vi "DP I-O Main Panel.vi"(11 "Expt State (in)":T2) -> (3 "State":T2)   [LabVIEW 2020]
uses:
  Typedefs/DP Stimulus Params.ctl
  epl-vi-lib/Utility VIs/Type Defs/Left-Right ring.ctl
  CFTS Main Panel SubVIs/CFTS-Experiment State.ctl
  Typedefs/DP-StimGen.ctl
  Typedefs/DP-Rejection Settings.ctl
  Typedefs/DP-Advanced Options.ctl
  CFTS Main Panel SubVIs/CFTS-Data Type Enum.ctl
panel:
  in  "Last user":string
  in  "Recalibrate":bool
  in  "Probe Mic Gain (dB)":dbl
  in  "Save Waves?":bool=TRUE
  out "User":string
  out "Run #":u16=14
  out "ID #":u16=1
  in  "Avg specs":T1={"# Time avgs "=8, "# Spectrum avgs"=4}
  out "Path":path
  in  "DP Params":T3={"Start (dB)"=20.0, "Stop (dB)"=70.0, "Step (dB)"=10.0, "Ear"=enum."Right", "Mode"=enum."L1 = L2 + 10 dB", "f2 freqs (kHz)"="5.6;8.0;11.3;16;22.6;32;"}
  out "advanced":bool
  in  "Advanced options":T5
  in  "Start":bool
  in  "Stop":bool
  out "exit signal":bool
  out "Error":bool
  in  "Reject":T6 caption="Rejection"
  in  "StimGen":T7={"Sampling Rate (Hz)"=200000.0, "Npts"=10000, "Data Folder"=path "", "Acoustic System"="", "Recalibrate?"=FALSE, "AO Channels"=[], "Mic  gain (dB)"=0.0, "F1, F2 speakers"=[], "Override recal check"=FALSE}
  out "Freqs":cluster{"f1":dbl, "f2":dbl, "2f1-f2":dbl}={"f1"=9419.759114583332, "f2"=11291.50390625, "2f1-f2"=7548.014322916664} {"2f1-f2" format="%.3f"; "f1" format="%.3f"; "f2" format="%.3f"}
  out "Abort":bool
  out "running":bool
  out "DP window":cluster{i32, "df (Hz)":dbl, dbl[]}(graph)={0, "df (Hz)"=0.02, []}
  out "I-O Plot":cluster{cluster{dbl, dbl}[]}[](graph)
  in  "Notes":string
  out "Full Spectrum":cluster{i32, "Freq Resolution":dbl, dbl[]}(graph)={0, "Freq Resolution"=20.345052083333332, []}
  in  "RETURN":bool
  # "Stimulus"
  # "Averaging"
  # "Response"
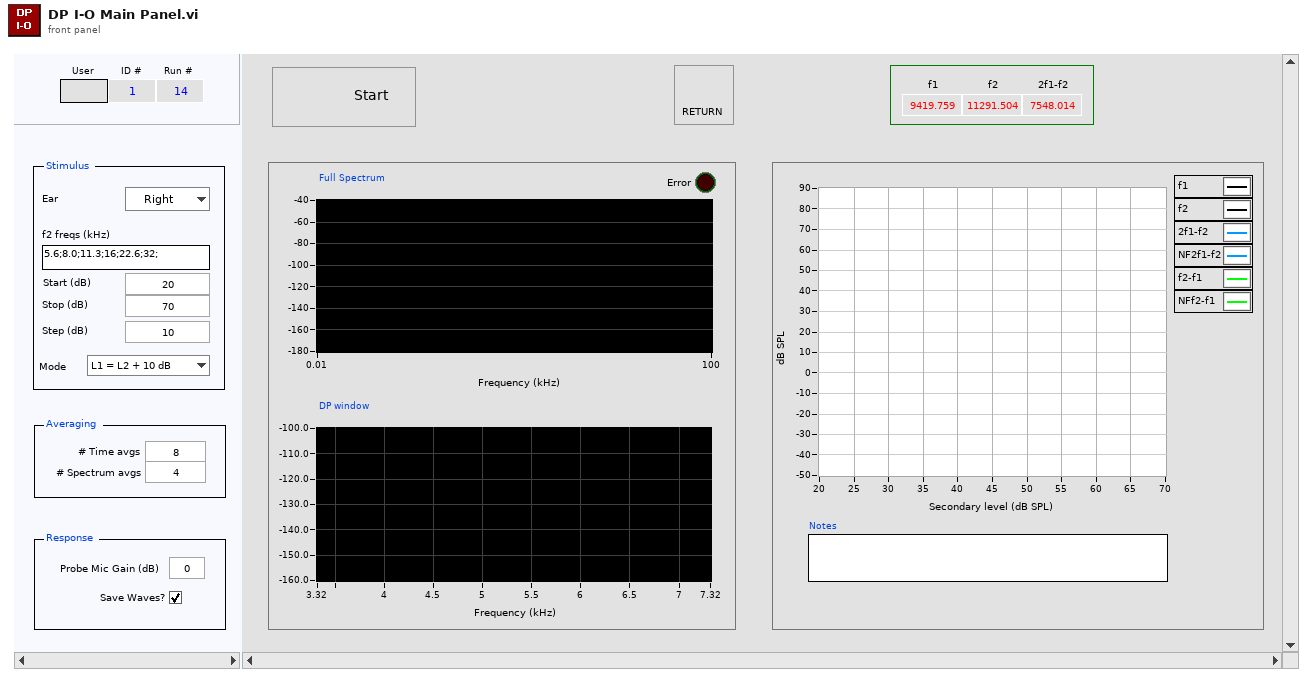
[diagram p1: front panel]
types:
  T1 = cluster{"# Time avgs ":i32, "# Spectrum avgs":i32}
  T2 = typedef "CFTS-Experiment State.ctl" = cluster{"Experimenter":string, "Number":u32, "Right":string, "Left":string, "Data Folder":path, "State File":path, "Version Info":string, "End Exposure Time":dbl, "Exposure Duration":string, "Run #":cluster{"CAP":i16, "ABR":i16, "DP":i16, "VsEP":i16, "MeasSeq":i16, "SubSeq":i16, "SFOAE":i16}}
  T3 = typedef "DP Stimulus Params.ctl" = cluster{"Start (dB)":dbl, "Stop (dB)":dbl, "Step (dB)":dbl, "Ear":T4, "Mode":enum16{"L1 = L2", "L1 = L2 + 10 dB"}, "f2 freqs (kHz)":string}
  T4 = typedef "Left-Right ring.ctl" = enum16{"Right", "Left"}
  T5 = typedef "DP-Advanced Options.ctl" = cluster{"TimeAvgExpr":string, "FreqAvgExpr":string}
  T6 = typedef "DP-Rejection Settings.ctl" = cluster{"Override":bool, "dB re 2f1-f2":dbl, "Min (dB SPL)":dbl}
  T7 = typedef "DP-StimGen.ctl" = cluster{"Sampling Rate (Hz)":dbl, "Npts":i32, "Data Folder":path, "Acoustic System":string, "Recalibrate?":bool, "AO Channels":i32[], "Mic  gain (dB)":dbl, "F1, F2 speakers":i32[], "Override recal check":bool}
  T8 = typedef "CFTS-Data Type Enum.ctl" = enum16{"CAP", "ABR", "DP", "VsEP", "MeasSeq", "SFOAE"}
  T9 = typedef "DP-Freqs.ctl" = cluster{"f1":dbl, "f2":dbl, "2f1-f2":dbl}
  T10 = typedef "DP-DataAcq.ctl" = cluster{"#spectra avgs":i32[], "#time avgs":i32[], "dt (ms)":dbl, "df (kHz)":dbl, "Npts":i32, "Save waves?":bool, "Data File":path, "AI Channels":u16[], "Sampling rate (Hz)":dbl, "Probe Tube Sensitivity":cluster{"Frequency":dbl[], "Mag":dbl[]}, "Mic gain (dB)":dbl, "ptIndex":i32}
  T11 = typedef "CFTS-Options.ctl" = cluster{"DP Artifact Rejection":bool, "Monitor vital signs ":bool, "Extension":string}
  T12 = cluster{"Shift":bool, "Ctrl":bool, "Alt":bool, "Cmd":bool, "Opt":bool}
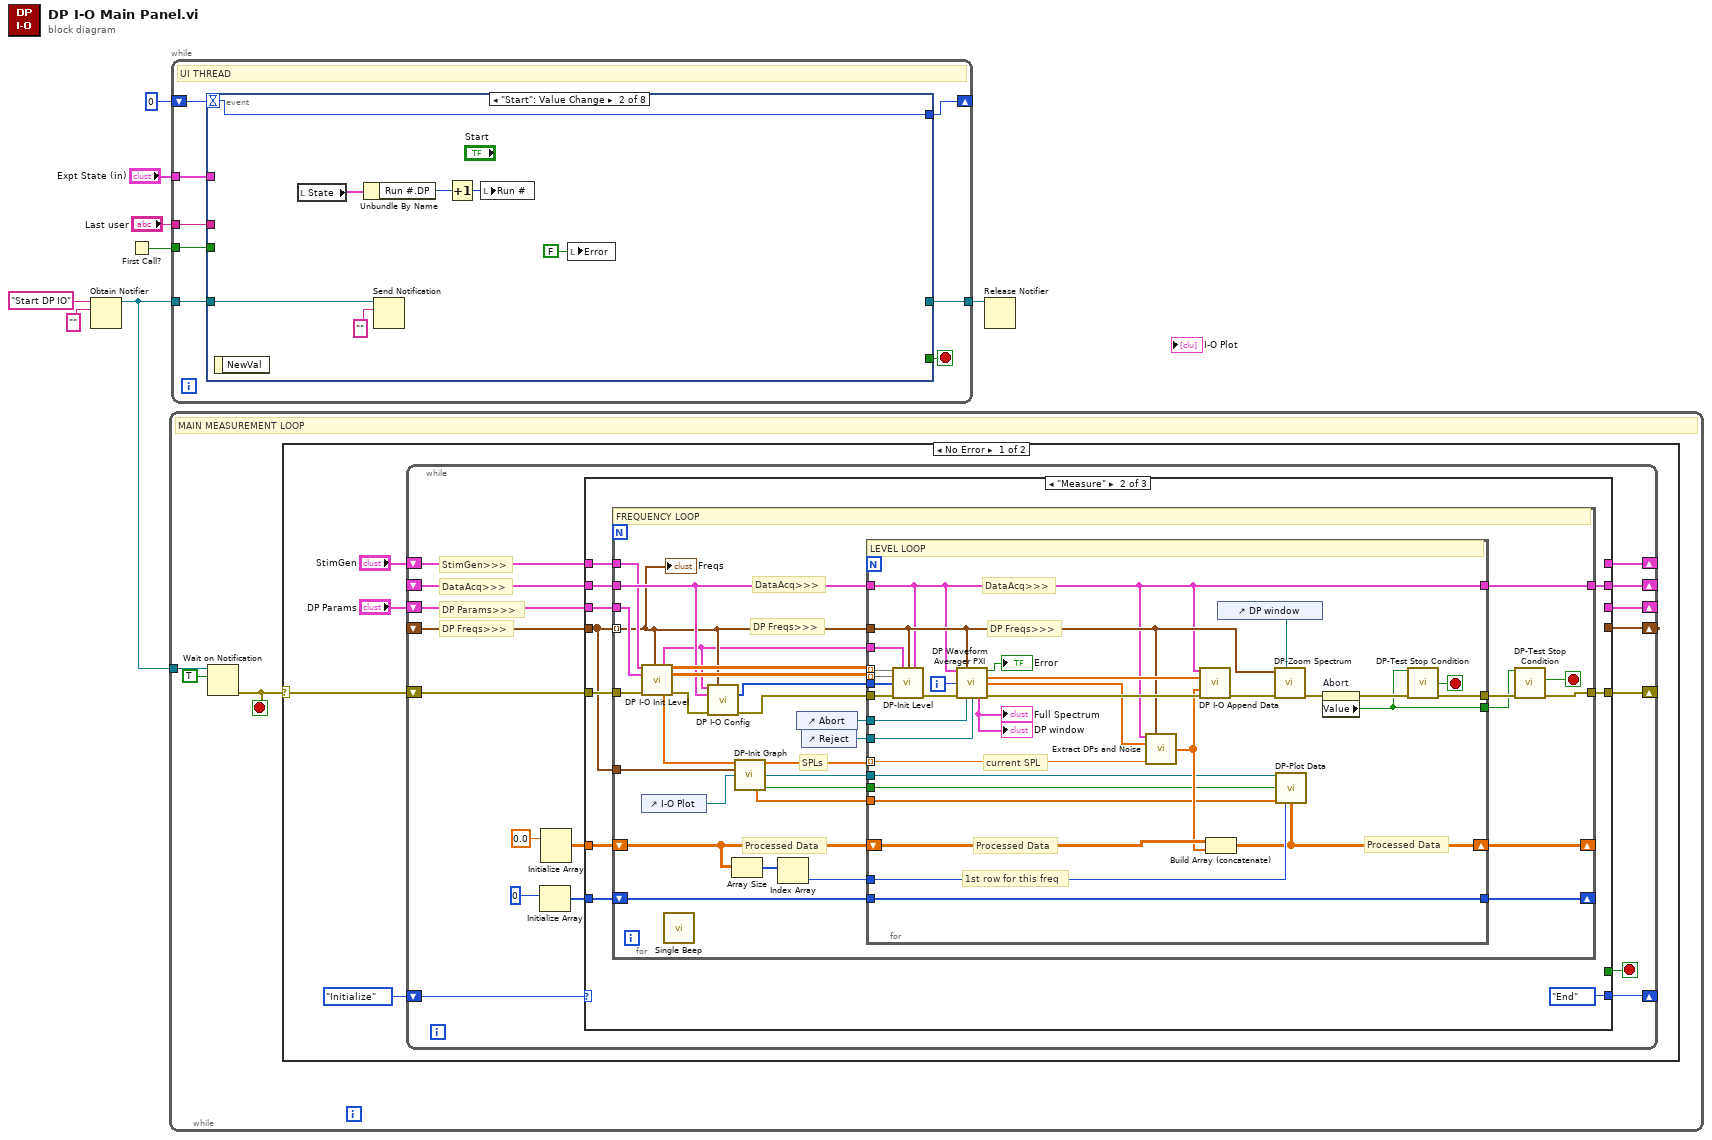
[diagram p0: block diagram]
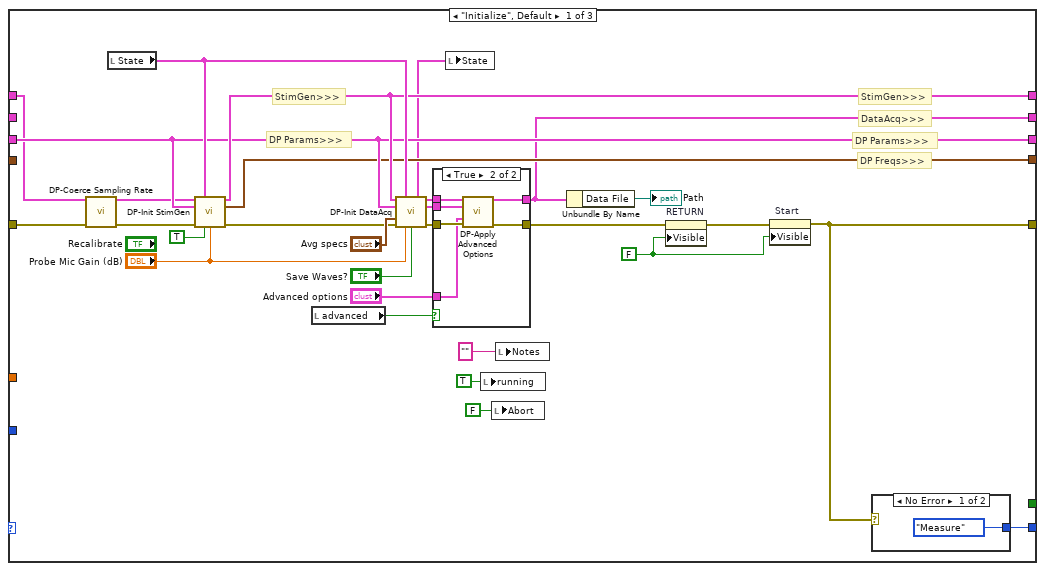
[diagram p2: hidden frame]
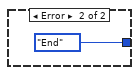
[diagram p4: hidden frame]
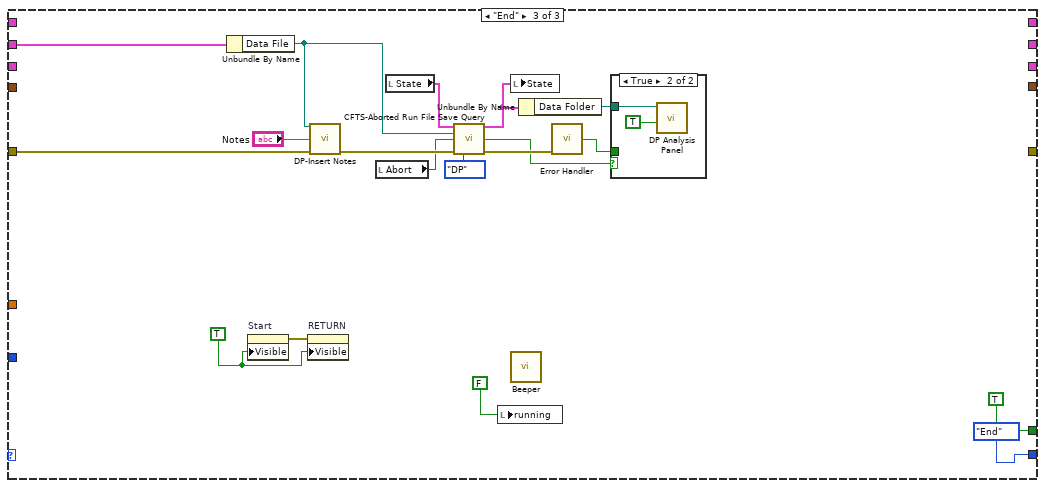
[diagram p5: hidden frame]
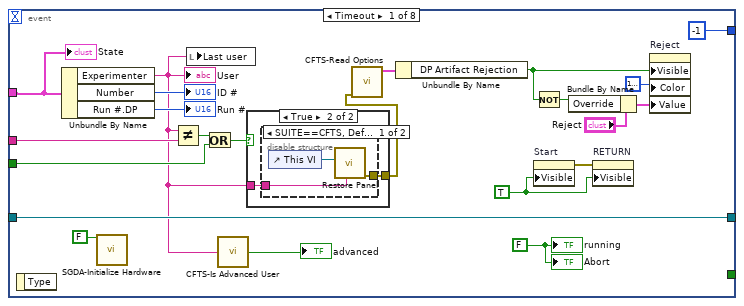
[diagram p8: hidden frame]
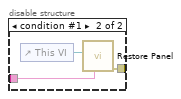
[diagram p10: hidden frame]
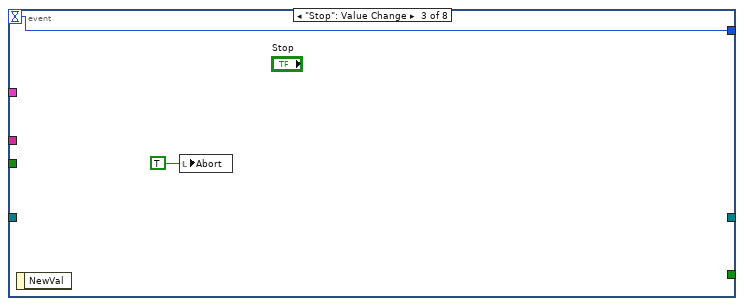
[diagram p11: hidden frame]
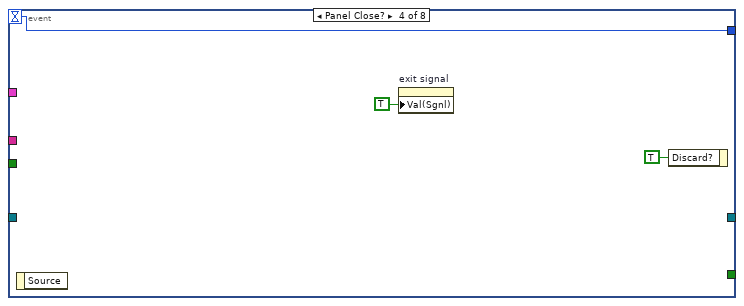
[diagram p12: hidden frame]
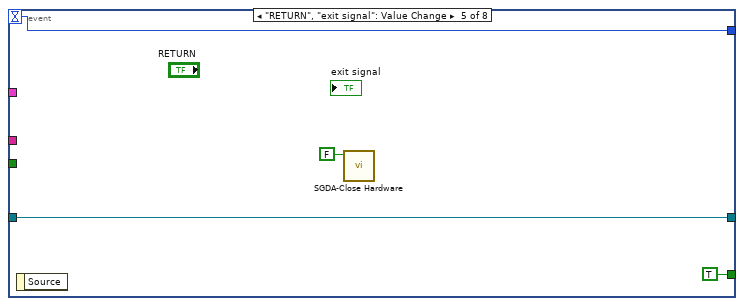
[diagram p13: hidden frame]
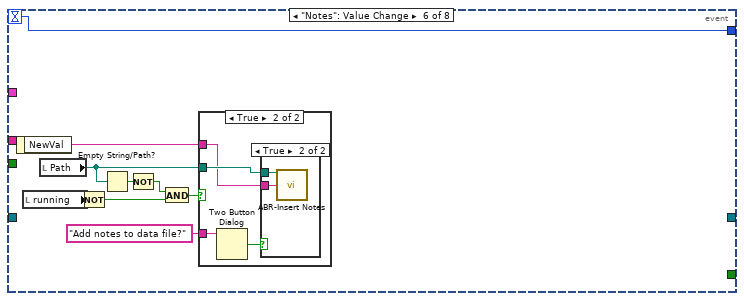
[diagram p14: hidden frame]
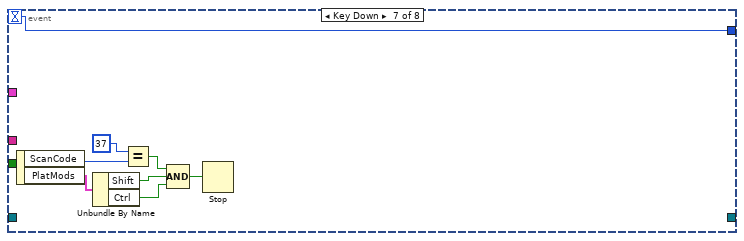
[diagram p17: hidden frame]
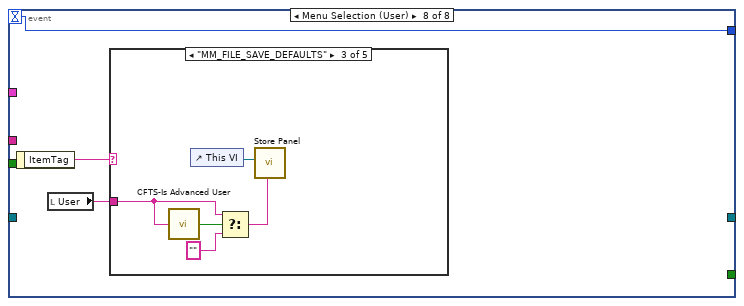
[diagram p18: hidden frame]
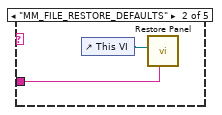
[diagram p20: hidden frame]
diagram:
  n1 = Obtain Notifier(name (unnamed)="Start DP IO", notification data type="") -> (notifier out=w8:refnum<notifier>)  [unwired: 2 in, 2 out]
  n2 = First Call?() -> (First Call?: T/F=w3:bool)
  n3 = while {
    tunnel: w8 -> [w10]
    stop <- w9 stop-if-true
    # "MAIN MEASUREMENT LOOP"
    n4 = Wait on Notification(notifier=w10, ignore previous (F)=TRUE) -> (error out=w9:errorcluster)  [unwired: 2 in, 3 out]
    n5 = case shown="No Error" w9 {
      selector: w9 -> [w12 _]
      frame No Error {
        n6 = while {
          shift-right: [w31] -> _
          shift-left: w12 -> [w32]
          shift-right: [w22] -> _
          shift-left: enum16{"Initialize", "Measure", "End"}."Initialize" -> [w30]
          shift-right: [w26] -> _
          shift-left: "StimGen" -> [w28]
          shift-right: [w25] -> _
          shift-left: _ -> [w27]
          shift-right: [w23] -> _
          shift-left: "DP Params" -> [w24]
          shift-right: [w21] -> _
          shift-left: _ -> [w20]
          stop <- w29 stop-if-true
          # "DP Freqs>>>"
          # "DP Params>>>"
          # "DataAcq>>>"
          # "StimGen>>>"
          n7 = Initialize Array(0) -> (w16:i32[])  [unwired: 1 in]
          n8 = Initialize Array(0.0) -> (w18:dbl[][])  [unwired: 2 in]
          n9 = case shown="\"Measure\"" w30 {
            tunnel: w32 -> [w36 w81 w154]
            tunnel: [w46 w80 _] -> w31
            tunnel: [_ _ TRUE] -> w29
            tunnel: w28 -> [w34 w78 _]
            tunnel: w27 -> [_ w76 w155]
            tunnel: [w54 _ _] -> w26
            tunnel: [w42 w74 _] -> w25
            tunnel: w24 -> [w51 w77 _]
            tunnel: [w51 _ _] -> w23
            tunnel: [w45 enum16{"Initialize", "Measure", "End"}."End" enum16{"Initialize", "Measure", "End"}."End"] -> w22
            tunnel: [w50 _ _] -> w21
            tunnel: w20 -> [_ w73 _]
            tunnel: w18 -> [_ w79 _]
            tunnel: w16 -> [_ w72 _]
            frame "Initialize", Default {
              w58 = FALSE
              # "DP Freqs>>>"
              # "DP Params>>>"
              # "StimGen>>>"
              # "DP Params>>>"
              # "DataAcq>>>"
              # "StimGen>>>"
              n10 = call "DP-Coerce Sampling Rate.vi"("StimGen (out) in"=w34, "error in (no error)"=w36) -> ("StimGen (out) out"=w33:T7, "error out"=w35:errorcluster)  [unwired: 12 in]
              n11 = local read "State"() -> (w55:T2)
              n12 = call "DP-Init StimGen.vi"("StimGen"=w33, "Expt State"=w55, "DP stimulus params"=w51, "error in (no error)"=w35, "Recalibrate?"=TRUE, "Mic  gain (dB)"="Probe Mic Gain (dB)") -> ("StimGen (out)"=w54:T7, "DP Freqs"=w50:T9[], "error out"=w53:errorcluster)  [unwired: 7 in]
              n13 = local read "advanced"() -> (w39:bool)
              n14 = call "DP-Init DataAcq.vi"("StimGen"=w54, "Expt State"=w55, "DP stimulus params"=w51, "Avg specs"="Avg specs", "error in (no error)"=w53, "Mic gain (dB)"="Probe Mic Gain (dB)", "Save waves?"="Save Waves?") -> ("Expt State out"=w48:T2, "DataAcq"=w41:T10, "DP thru"=w37:T3, "error out"=w43:errorcluster)  [unwired: 5 in]
              n15 = case shown="True" w39 {
                tunnel: w43 -> [w62 w68]
                tunnel: [w63 w67] -> w42
                tunnel: w41 -> [w63 w69]
                tunnel: [w62 w66] -> w40
                tunnel: "Advanced options" -> [_ w65]
                tunnel: w37 -> [_ w64]
                frame False {
                }
                frame True {
                  n16 = call "DP-Apply Advanced Options.vi"("DataAcq in"=w69, "DP params"=w64, "Advanced options"=w65, "error in (no error)"=w68) -> ("DataAcq out"=w67:T10, "error out"=w66:errorcluster)  [unwired: 10 in]
                }
              }
              n17 = local write "State"(w48) -> ()
              n18 = local write "running"(TRUE ("running")) -> ()
              n19 = local write "Abort"(FALSE ("Stopping")) -> ()
              n20 = local write "Notes"("" ("Notes")) -> ()
              n21 = Unbundle By Name(w42) -> ("Data File"=→"Path":path)
              n22 = property on="RETURN" class="Bool"(error in=w40, "Visible"=w58) -> (error out=w52:errorcluster)  [unwired: 1 in, 1 out]
              n23 = property on="Start" class="Bool"(error in=w52, "Visible"=w58) -> (error out=w46:errorcluster)  [unwired: 1 in, 1 out]
              n24 = case shown="No Error" w46 {
                tunnel: [enum16{"Initialize", "Measure", "End"}."Measure" enum16{"Initialize", "Measure", "End"}."End"] -> w45
                frame No Error {
                }
                frame Error {
                }
              }
            }
            frame "Measure" {
              n25 = for {
                shift-right: [w104] -> _
                shift-left: w79 -> [w110]
                tunnel: w81 -> [w107]
                tunnel: [w97] -> w80
                tunnel: w73 -> [w92] mode=indexing
                tunnel: w78 -> [w93]
                tunnel: w77 -> [w103]
                tunnel: w76 -> [w101]
                tunnel: [w100] -> w74
                tunnel: w73 -> [w87]
                shift-right: [w90] -> _
                shift-left: w72 -> [w91]
                stop <- w102 stop-if-true
                # "DP Freqs>>>"
                # "DataAcq>>>"
                # "Processed Data"
                # "SPLs"
                # "FREQUENCY LOOP"
                n26 = call "DP I-O Init Level.vi"("StimGen"=w93, "DP Freqs"=w92, "DP stimulus params"=w103, "error in (no error)"=w107) -> ("StimGen Out"=w82:T7, "Multipliers (2D)"=w112:dbl[][], "Gains (2D)"=w111:dbl[][], "Nominal f2 SPL"=w89:dbl[], "error out"=w106:errorcluster)  [unwired: 5 in, 2 out]
                n27 = control-ref of="I-O Plot"() -> (w86:refnum<vi>)
                n28 = call "Single Beep.vi"() -> ()  [unwired: 1 in]
                n29 = call "DP I-O Config.vi"("StimGen"=w82, "DP Freqs"=w92, "DataAcq"=w101, "error in (no error)"=w106) -> ("AO Channels"=w99:i32[], "error out"=w105:errorcluster)  [unwired: 10 in]
                n30 = Array Size(array=w110) -> (size(s)=w109:i32[])
                n31 = call "DP-Init Graph.vi"("Nominal f2 SPL in"=w89, "DP Freqs"=w87, "XYGraph in"=w86) -> ("Nominal f2 SPL out"=w88:dbl[], "XYGraph out"=w85:refnum<vi>, "f2"=w83:dbl[], "plot vs freq"=w84:bool)  [unwired: 9 in]
                n32 = Index Array(array=w109) -> (element=w108:i32)  [unwired: 1 in]
                n33 = control-ref of="Abort"() -> (w95:refnum<vi>)
                n34 = control-ref of="Reject"() -> (w94:refnum<vi>)
                n35 = for {
                  tunnel: w112 -> [w118] mode=indexing
                  tunnel: w111 -> [w117] mode=indexing
                  tunnel: w88 -> [w135] mode=indexing
                  shift-right: [w120] -> w104
                  shift-left: w110 -> [w143]
                  tunnel: w108 -> [w122]
                  tunnel: w105 -> [w144]
                  tunnel: [w132] -> w98
                  tunnel: w101 -> [w113]
                  tunnel: w92 -> [w114]
                  tunnel: [w113] -> w100
                  tunnel: w99 -> [w116]
                  tunnel: [w129] -> w96
                  tunnel: w95 -> [w128]
                  tunnel: w94 -> [w127]
                  tunnel: w91 -> [w125]
                  tunnel: [w125] -> w90
                  tunnel: w85 -> [w124]
                  tunnel: w84 -> [w123]
                  tunnel: w83 -> [w121]
                  tunnel: w82 -> [w115]
                  i -> [w119]
                  stop <- w141 stop-if-true
                  # "DP Freqs>>>"
                  # "DataAcq>>>"
                  # "current SPL"
                  # "1st row for this freq"
                  # "Processed Data"
                  # "Processed Data"
                  # "LEVEL LOOP"
                  n36 = call "DP-Init Level.vi"("Multipliers (2D)"=w118, "StimGen Out"=w115, "DP Freqs"=w114, "DataAcq in"=w113, "Gains (2D)"=w117, "AO Channels"=w116, "error in (no error)"=w144) -> ("error out"=w140:errorcluster)  [unwired: 8 in]
                  n37 = call "DP Waveform Averager PXI.vi"("DataAcq"=w113, "DP Freqs"=w114, "iLevel"=w119, "error in"=w140, "Abort"=w128, "Reject Ref"=w127) -> ("Error?"=→"Error":bool, "Ave Wave"=w134:dbl[], "Averaged Spectrum (Vrms)"=w137:dbl[], "waveform cluster"=→"Full Spectrum" →"DP window":cluster{i32, "dx":dbl, "Array":dbl[]}, "error out"=w139:errorcluster)  [unwired: 4 in, 1 out]
                  n38 = call "Extract DPs and Noise.vi"("DataAcq"=w113, "DP Freqs"=w114, "Spectrum in Vrms"=w137, "SPL"=w135) -> ("Output Array"=w136:dbl[])  [unwired: 11 in]
                  n39 = call "DP I-O Append Data.vi"("DataAcq"=w113, "Waveform"=w134, "Processed data"=w136, "error in (no error)"=w139) -> ("error out"=w142:errorcluster)  [unwired: 11 in]
                  n40 = Build Array (concatenate)(w143, w136) -> (w120:dbl[][])
                  n41 = control-ref of="DP window"() -> (w133:refnum<vi>)
                  n42 = call "DP-Zoom Spectrum.vi"("DP window"=w133, "error in (no error)"=w142, "DP Freqs"=w114) -> ("error out"=w131:errorcluster)  [unwired: 8 in]
                  n43 = call "DP-Plot Data.vi"("XYGraph"=w124, "vs Freq"=w123, "f2"=w121, "1st row current freq"=w122, "Input Array (4xn)"=w120) -> ()  [unwired: 11 in]
                  n44 = property on="Abort" class="Bool (strict)"(error in=w131) -> (error out=w130:errorcluster, "Value"=w129:bool)  [unwired: 1 in, 1 out]
                  n45 = call "DP-Test Stop Condition.vi"("Abort?"=w129, "error in (no error)"=w130) -> ("Stop?"=w141:bool, "error out"=w132:errorcluster)  [unwired: 12 in]
                }
                n46 = call "DP-Test Stop Condition.vi"("Abort?"=w96, "error in (no error)"=w98) -> ("Stop?"=w102:bool, "error out"=w97:errorcluster)  [unwired: 12 in]
                "Freqs" <- w92
              }
            }
            frame "End" {
              w161 = TRUE
              n47 = Unbundle By Name(w155) -> ("Data File"=w151:path)
              n48 = property on="Start" class="Bool"("Visible"=w161) -> (error out=w157:errorcluster)  [unwired: 2 in, 1 out]
              n49 = property on="RETURN" class="Bool"(error in=w157, "Visible"=w161) -> ()  [unwired: 1 in, 2 out]
              n50 = call "DP-Insert Notes.vi"("path"=w151, "Notes"="Notes", "error in (no error)"=w154) -> ("error out"=w156:errorcluster)  [unwired: 12 in]
              n51 = local read "Abort"() -> (w149:bool)
              n52 = local read "State"() -> (w152:T2)
              n53 = call "CFTS-Aborted Run File Save Query.vi"("Expt State"=w152, "Path"=w151, "Aborted"=w149, "error in (no error)"=w156, "Data Type"=CFTS-Data_Type_Enum."DP") -> ("Expt State out"=w148:T2, "File saved?"=w146:bool, "error out"=w153:errorcluster)  [unwired: 8 in]
              n54 = local write "running"(FALSE ("running")) -> ()
              n55 = local write "State"(w148) -> ()
              n56 = call "Beeper.vi"() -> ()  [unwired: 5 in, 1 out]
              n57 = Unbundle By Name(w148) -> ("Data Folder"=w147:path)
              n58 = call "Error Handler.vi"("error in (no error)"=w153) -> ("error?"=w145:bool)  [unwired: 13 in, 1 out]
              n59 = case shown="True" w146 {
                tunnel: w147 -> [_ w164]
                tunnel: w145 -> [_ _]
                frame False {
                }
                frame True {
                  n60 = call "DP Analysis Panel.vi"("Autosave? (F)"=TRUE, "Data folder in"=w164) -> ()  [unwired: 10 in]
                }
              }
            }
          }
        }
      }
      frame Error {
      }
    }
  }
  n61 = while {
    tunnel: w8 -> [w172]
    shift-right: [w169] -> _
    shift-left: 0 -> [w170]
    tunnel: [w168] -> w4
    tunnel: w3 -> [w167]
    tunnel: "Expt State (in)" -> [w166]
    tunnel: "Last user" -> [w165]
    stop <- w171 stop-if-true
    # "UI THREAD"
    n62 = event shown="[1] \"Start\": Value Change" {
      selector: _ -> [_ _ _ _ _ _ _ _]
      dyn-events: _ -> [_ _ _ _ _ _ _ _]
      timeout: w170 -> [_ w204 w211 w214 w217 w219 w241 w244]
      tunnel: w172 -> [w188 w209 _ _ w216 _ _ _]
      tunnel: [_ _ _ _ TRUE _ _ _] -> w171
      tunnel: [-1 w204 w211 w214 w217 w219 w241 w244] -> w169
      tunnel: [w188 _ _ _ w216 _ _ _] -> w168
      tunnel: w167 -> [w178 _ _ _ _ _ _ _]
      tunnel: w166 -> [w181 _ _ _ _ _ _ _]
      tunnel: w165 -> [w180 _ _ _ _ _ _ _]
      event Timeout {
        w191 = TRUE
        w190 = FALSE ("quitting")
        n63 = event-data() -> ()  [unwired: 1 in, 1 out]
        n64 = Unbundle By Name(w181) -> ("Experimenter"=w174:string, "Number"=→"ID #":u32, "Run #.DP"=→"Run #":i16)
        "User" <- w174
        n65 = call "SGDA-Initialize Hardware.vi"("Start PXI Server"=FALSE) -> ()  [unwired: 13 in, 2 out]
        n66 = Not Equal?(x=w174, y=w180) -> (x != y?=w179:bool)
        n67 = local write "Last user"(w174) -> ()
        n68 = Or(x=w179, y=w178) -> (x .or. y?=w177:bool)
        n69 = call "CFTS-Is Advanced User.vi"("Experimenter"=w174) -> ("Advanced user"=→"advanced":bool)
        n70 = case shown="True" w177 {
          tunnel: w174 -> [_ w196]
          tunnel: [_ w195] -> w176
          frame False {
          }
          frame True {
            n71 = disable-structure shown="SUITE==CFTS, Default" {
              disable-tunnel: w196 -> [w198 w201]
              disable-tunnel: [w197 w200] -> w195
              frame condition #0 (active) {
                n72 = control-ref of="This VI"() -> (w199:refnum<vi>)
                n73 = call "Restore Panel.vi"("User"=w198, "VI reference"=w199) -> ("error out"=w197:errorcluster)  [unwired: 9 in]
              }
              frame condition #1 {
                n74 = control-ref of="This VI"() -> (w202:refnum<vi>)
                n75 = call "Restore Panel.vi"("User"=w201, "VI reference"=w202) -> ("error out"=w200:errorcluster)  [unwired: 9 in]
              }
            }
          }
        }
        n76 = call "CFTS-Read Options.vi"("error in (no error)"=w176) -> ("CFTS Options"=w187:T11)  [unwired: 9 in, 1 out]
        n77 = Unbundle By Name(w187) -> ("DP Artifact Rejection"=w183:bool)
        n78 = Not(x=w183) -> (.not. x?=w184:bool)
        n79 = property on="Start" class="Bool"("Visible"=w191) -> (error out=w189:errorcluster)  [unwired: 2 in, 1 out]
        n80 = Bundle By Name(cluster="Reject", "Override"=w184) -> (w182:T6)
        n81 = property on="RETURN" class="Bool"(error in=w189, "Visible"=w191) -> ()  [unwired: 1 in, 2 out]
        n82 = property on="Reject" class="Clust (strict)"("Visible"=w183, "Color"=u32 16777238, "Value"=w182) -> ()  [unwired: 2 in, 2 out]
        "State" <- w181
        "running" <- w190
        "Abort" <- w190
      }
      event "Start": Value Change {
        n83 = event-data() -> ()  [unwired: 1 in, 1 out]
        n84 = local read "State"() -> (w206:T2)
        n85 = Unbundle By Name(w206) -> ("Run #.DP"=w205:i16)
        n86 = Send Notification(notification="", notifier=w209) -> ()  [unwired: 1 in, 2 out]
        n87 = Increment(x=w205) -> (x+1=w207:i16)
        n88 = local write "Run #"(w207) -> ()
        n89 = local write "Error"(FALSE ("Error")) -> ()
      }
      event "Stop": Value Change {
        n90 = event-data() -> ()  [unwired: 1 in, 1 out]
        n91 = local write "Abort"(TRUE ("Stopping")) -> ()
      }
      event Panel Close? {
        n92 = event-data() -> ()  [unwired: 1 in, 1 out]
        n93 = property on="exit signal" class="Bool (strict)"("Val(Sgnl)"=TRUE ("Value (Signaling)")) -> ()  [unwired: 2 in, 2 out]
        n94 = event-data("Discard?"=TRUE) -> ()  [unwired: 1 in, 1 out]
      }
      event "RETURN", "exit signal": Value Change {
        n95 = event-data() -> ()  [unwired: 1 in, 1 out]
        n96 = call "SGDA-Close Hardware.vi"("Stop PXI Server (T)"=FALSE) -> ()  [unwired: 6 in, 1 out]
      }
      event "Notes": Value Change {
        n97 = event-data() -> ("NewVal"=w222:string)  [unwired: 1 in]
        n98 = local read "running"() -> (w220:bool)
        n99 = local read "Path"() -> (w221:path)
        n100 = Not(x=w220) -> (.not. x?=w224:bool)
        n101 = Empty String/Path?(string/path=w221) -> (empty?=w223:bool)
        n102 = Not(x=w223) -> (.not. x?=w225:bool)
        n103 = And(x=w225, y=w224) -> (x .and. y?=w226:bool)
        n104 = case shown="True" w226 {
          tunnel: w221 -> [_ w231]
          tunnel: w222 -> [_ w230]
          tunnel: "Add notes to data file?" ("message") -> [_ w229]
          frame False {
          }
          frame True {
            n105 = Two Button Dialog(message=w229) -> (T button?=w228:bool)  [unwired: 2 in]
            n106 = case shown="True" w228 {
              tunnel: w231 -> [_ w233]
              tunnel: w230 -> [_ w232]
              frame False {
              }
              frame True {
                n107 = call "ABR-Insert Notes.vi"("path"=w233, "Notes"=w232) -> ()  [unwired: 12 in, 2 out]
              }
            }
          }
        }
      }
      event Key Down {
        n108 = event-data() -> ("ScanCode"=w240:i16, "PlatMods"=w238:T12)  [unwired: 1 in]
        n109 = Unbundle By Name(w238) -> ("Shift"=w236:bool, "Ctrl"=w235:bool)
        n110 = Equal?(x=i16 37 ("y"), y=w240) -> (x = y?=w237:bool)
        n111 = Compound Arithmetic op=AND(w237, w236, w235) -> (w234:bool)
        n112 = Stop(stop? (T)=w234) -> ()
      }
      event Menu Selection (User) {
        n113 = event-data() -> ("ItemTag"=w243:string)  [unwired: 1 in]
        n114 = local read "User"() -> (w242:string)
        n115 = case shown="\"MM_FILE_SAVE_DEFAULTS\"" w243 {
          tunnel: w242 -> [_ w245 w249 _ _]
          frame "False", Default {
          }
          frame "MM_FILE_RESTORE_DEFAULTS" {
            n116 = control-ref of="This VI"() -> (w246:refnum<vi>)
            n117 = call "Restore Panel.vi"("User"=w245, "VI reference"=w246) -> ()  [unwired: 9 in, 1 out]
          }
          frame "MM_FILE_SAVE_DEFAULTS" {
            n118 = call "CFTS-Is Advanced User.vi"("Experimenter"=w249) -> ("Advanced user"=w250:bool)
            n119 = control-ref of="This VI"() -> (w251:refnum<vi>)
            n120 = Select(t=w249, s=w250, f="") -> (s? t:f=w248:string)
            n121 = call "Store Panel.vi"("User"=w248, "VI reference"=w251) -> ()  [unwired: 9 in, 1 out]
          }
          frame "MM_FILE_OPTIONS" {
            n122 = local read "Advanced options"() -> (w255:T5)
            n123 = local read "advanced"() -> (w253:bool)
            n124 = control-ref of="This VI"() -> (w252:refnum<vi>)
            n125 = local read "StimGen"() -> (w257:T7)
            n126 = call "DP-Options Dialog.vi"("Parent VI"=w252, "Advanced options"=w255, "StimGen"=w257, "Advanced?"=w253) -> ("Advanced options out"=w254:T5, "StimGen out"=w256:T7)  [unwired: 5 in, 1 out]
            n127 = local write "Advanced options"(w254) -> ()
            n128 = local write "StimGen"(w256) -> ()
          }
          frame "MM_FILE_EXIT" {
            n129 = property on="exit signal" class="Bool (strict)"("Val(Sgnl)"=TRUE ("Value (Signaling)")) -> ()  [unwired: 2 in, 2 out]
          }
        }
      }
    }
  }
  n130 = Release Notifier(notifier=w4) -> ()  [unwired: 2 in, 3 out]
